vi "Map XY.vi"(0 "Display State In":T2, 5 "XY":cluster{dbl, dbl}, 7 "plotnum":i32, 9 "Container State":T7, 11 "error in (no error)":errorcluster) -> (4 "Display State Out":T2, 6 "Coords":T1, 15 "error out":errorcluster)   [LabVIEW 2015, in "Interactive Graph.xctl"]
uses:
  Interactive Graph.xctl
  <vilib>/_xctls/Container State.ctl
  State.vi
  Persistent.ctl
  Plot.ctl
  EPhys/LV Source/Work Panel VIs/Typedefs/EPhysWork-Label Position.ctl
  Events.ctl
  Selection.ctl
  XRange.ctl
  YScale.ctl
  Cursor.ctl
  <vilib>/Utility/miscctls.llb/LVPoint32TypeDef.ctl
  <vilib>/_xctls/XControlSupport.lvlib
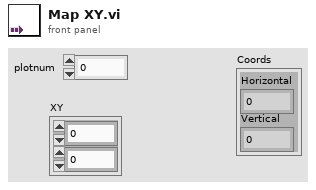
[diagram p1: front panel]
types:
  T1 = typedef "LVPoint32TypeDef.ctl" = cluster{"Horizontal":i32, "Vertical":i32}
  T2 = typedef "Interactive Graph.xctl/State.vi" = cluster{"ref":refnum<vi>, "actions":string[], "Persist":T3, "cursor":bool, "prescale":dbl, "palette":u32[], "colIndex":i32, "to add":T4, "Events":T6, "selected":i32, "to show":cluster{"Visible":bool, "Start":i32, "Length":i32}, "maxplot":i32, "Y0":dbl[], "plotnum":i32}
  T3 = typedef "Interactive Graph.xctl/Persistent.ctl" = cluster{"Scale":dbl, "Xrange":cluster{"min":dbl, "max":dbl}}
  T4 = typedef "Interactive Graph.xctl/Plot.ctl" = cluster{"plot":cluster{"X":dbl[], "Y":dbl[]}, "name":string, "Y0":dbl, "color":u32, "Style":enum16{"Normal", "Highlight", "Shadow"}, "labpos":T5, "visible":bool, "cursor":bool}
  T5 = typedef "EPhysWork-Label Position.ctl" = cluster{"Index":i32, "Xoff":dbl, "Yoff":dbl}
  T6 = typedef "Interactive Graph.xctl/Events.ctl" = cluster{"Selection":refnum<user-event>, "XRange":refnum<user-event>, "YScale":refnum<user-event>, "CursorPos":refnum<user-event>}
  T7 = typedef "XControlSupport.lvlib/Container State.ctl" = cluster{"Indicator?":bool, "Run Mode?":bool, " Refnum":refnum<vi>}
  T8 = typedef "LVRectTypeDef.ctl" = cluster{"Left":i16, "Top":i16, "Right":i16, "Bottom":i16}
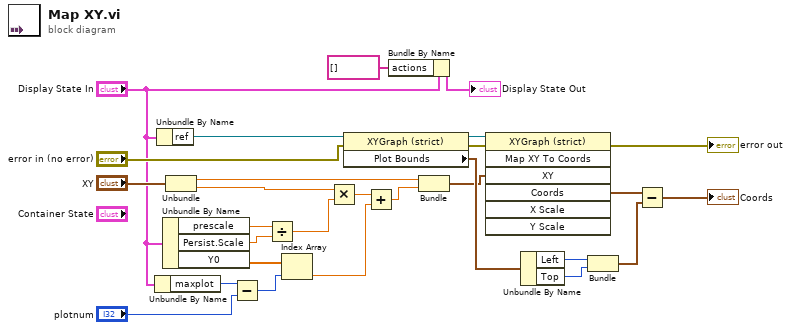
[diagram p0: block diagram]
diagram:
  n1 = Unbundle By Name("Display State In") -> ("maxplot"=w15:i32)
  n2 = Unbundle By Name("Display State In") -> ("ref"=w26:refnum<vi>)
  n3 = Unbundle By Name("Display State In") -> ("prescale"=w12:dbl, "Persist.Scale"=w11:dbl, "Y0"=w9:dbl[])
  n4 = Unbundle("XY") -> (w2:dbl, w7:dbl)
  n5 = Subtract(x=w15, y="plotnum") -> (x-y=w8:i32)
  n6 = Divide(x=w12, y=w11) -> (x/y=w6:dbl)
  n7 = Index Array(array=w9, index=w8) -> (element=w4:dbl)
  n8 = Multiply(x=w7, y=w6) -> (x*y=w5:dbl)
  n9 = property class="XYGraph (strict)"(reference=w26, error in="error in (no error)") -> (reference out=w24:refnum<vi>, error out=w23:errorcluster, "Plot Bounds"=w19:T8)
  n10 = Add(x=w5, y=w4) -> (x+y=w3:dbl)
  n11 = Bundle By Name(cluster="Display State In", "actions"=string[] []) -> (→"Display State Out":T2)
  n12 = Bundle(w2, w3) -> (w1:cluster{dbl, dbl})  [unwired: 1 in]
  n13 = invoke class="XYGraph (strict)" method="Map XY To Coords"(reference=w24, error in=w23, "XY"=w1) -> (error out=→"error out":errorcluster, "Coords"=w16:T1)  [unwired: 4 in, 5 out]
  n14 = Unbundle By Name(w19) -> ("Left"=w20:i16, "Top"=w21:i16)
  n15 = Bundle("Left"=w20, "Top"=w21) -> (w18:cluster{"Left":i16, "Top":i16})  [unwired: 1 in]
  n16 = Subtract(x=w16, y=w18) -> (x-y=→"Coords":T1)
